vi "Trim_Scan_List.vi"(8 "error in":errorcluster, 11 "DAQ970 in":refnum<class "DAQ970.lvclass">) -> (0 "error out":errorcluster, 3 "DAQ970 out":refnum<class "DAQ970.lvclass">)   [LabVIEW 2019, in "DAQ970.lvlib" / "DAQ970.lvclass"]
uses:
  Library/DAQ970.lvclass
  Library/DAQ970.lvclass/DAQ970.ctl
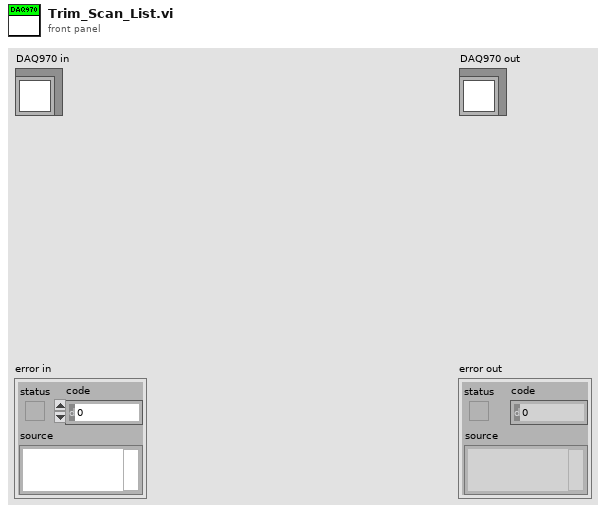
[diagram p1: front panel]
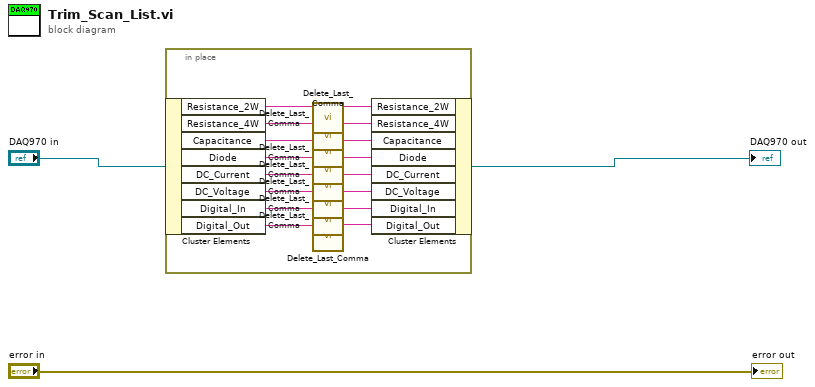
[diagram p0: block diagram]
diagram:
  n1 = in-place {
    n2 = in-place-cluster #1("DAQ970 in") -> ("Resistance_2W"=w19:string, "Resistance_4W"=w18:string, "Capacitance"=w17:string, "Diode"=w16:string, "DC_Current"=w15:string, "DC_Voltage"=w14:string, "Digital_In"=w13:string, "Digital_Out"=w5:string)
    n3 = call "Delete_Last_Comma.vi"("String"=w19) -> ("String 2"=w6:string)  [unwired: 10 in]
    n4 = call "Delete_Last_Comma.vi"("String"=w18) -> ("String 2"=w7:string)  [unwired: 10 in]
    n5 = call "Delete_Last_Comma.vi"("String"=w17) -> ("String 2"=w8:string)  [unwired: 10 in]
    n6 = call "Delete_Last_Comma.vi"("String"=w16) -> ("String 2"=w9:string)  [unwired: 10 in]
    n7 = call "Delete_Last_Comma.vi"("String"=w15) -> ("String 2"=w10:string)  [unwired: 10 in]
    n8 = call "Delete_Last_Comma.vi"("String"=w14) -> ("String 2"=w11:string)  [unwired: 10 in]
    n9 = call "Delete_Last_Comma.vi"("String"=w13) -> ("String 2"=w12:string)  [unwired: 10 in]
    n10 = call "Delete_Last_Comma.vi"("String"=w5) -> ("String 2"=w4:string)  [unwired: 10 in]
    n11 = in-place-cluster #1("Resistance_2W"=w6, "Resistance_4W"=w7, "Capacitance"=w8, "Diode"=w9, "DC_Current"=w10, "DC_Voltage"=w11, "Digital_In"=w12, "Digital_Out"=w4) -> (→"DAQ970 out":refnum<class "DAQ970.lvclass">)
  }
  "error out" <- "error in"
